vi "运维调试_古田户外.vi"() -> ()   [LabVIEW 2016]
uses:
  <vilib>/Utility/miscctls.llb/LVPointTypeDef.ctl
  PLC/PLC.lvlib
panel:
  in  "运维调试单选按钮":T1(xcontrol)
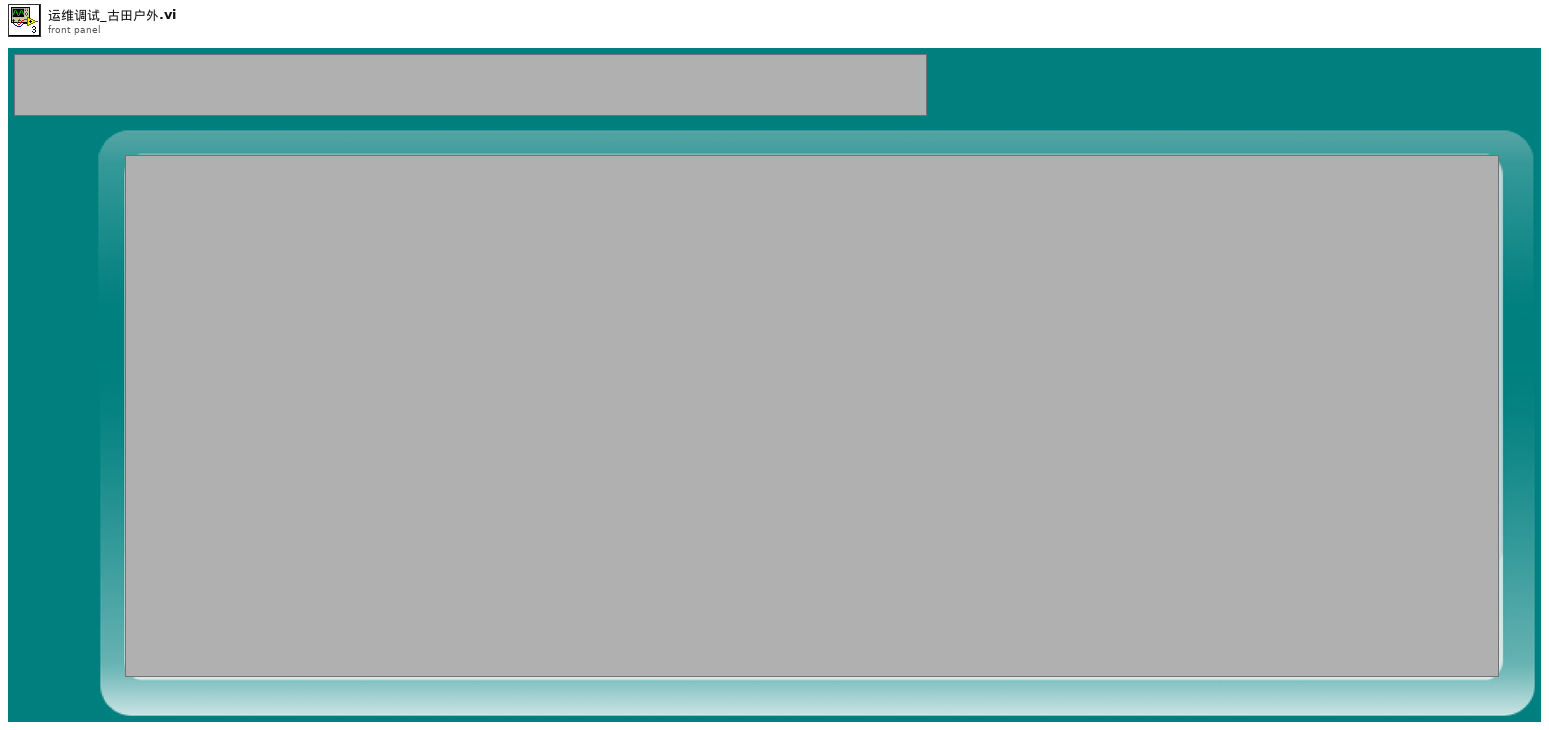
[diagram p1: front panel]
types:
  T1 = enum16{"采配水", "CODmn", "总磷氨氮", "多参数", "质控单元", "其他"}
  T2 = typedef "LVPointTypeDef.ctl" = cluster{"Horizontal":i16, "Vertical":i16}
  T3 = enum32{"Bad", "Idle", "Run top level", "Running"}
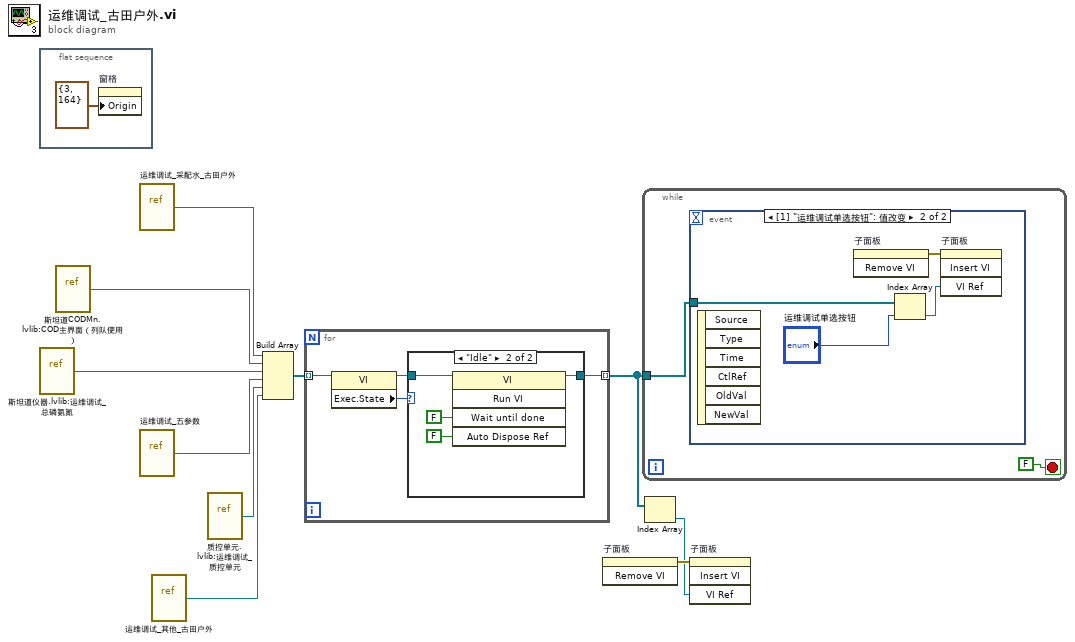
[diagram p0: block diagram]
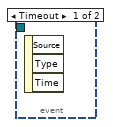
[diagram p3: hidden frame]
diagram:
  n1 = flat-sequence {
    frame #0 {
      n2 = property on="窗格" class="Pane"("Origin"=T2 {"Horizontal"=3, "Vertical"=164} ("原点")) -> ()  [unwired: 2 in, 2 out]
    }
  }
  n3 = vi-ref "斯坦道仪器.lvlib:运维调试_总磷氨氮.vi"() -> (w3:refnum<vi>)
  n4 = vi-ref "斯坦道CODMn.lvlib:COD主界面（列队使用）.vi"() -> (w4:refnum<vi>)
  n5 = vi-ref "运维调试_采配水_古田户外.vi"() -> (w7:refnum<vi>)
  n6 = vi-ref "运维调试_五参数.vi"() -> (w6:refnum<vi>)
  n7 = vi-ref "运维调试_其他_古田户外.vi"() -> (w2:refnum<vi>)
  n8 = vi-ref "质控单元.lvlib:运维调试_质控单元.vi"() -> (w1:refnum<vi>)
  n9 = Build Array(w7, w4, w3, w6, w1, w2) -> (w5:refnum<vi>[])
  n10 = for {
    tunnel: w5 -> [w15] mode=indexing
    tunnel: [w12] -> w9 mode=indexing
    n11 = property class="VI"(reference=w15) -> (reference out=w13:refnum<vi>, "Exec.State"=w14:T3)  [unwired: 1 in, 1 out]
    n12 = case shown="\"Idle\"" w14 {
      tunnel: w13 -> [w16 w18]
      tunnel: [w16 w17] -> w12
      frame "Bad", Default {
      }
      frame "Idle" {
        n13 = invoke class="VI" method="Run VI"(reference=w18, "Wait until done"=FALSE ("结束前等待"), "Auto Dispose Ref"=FALSE ("自动销毁引用")) -> (reference out=w17:refnum<vi>)  [unwired: 2 in, 4 out]
      }
    }
  }
  n14 = invoke on="子面板" class="SubPnl" method="Remove VI"() -> (error out=w10:errorcluster)  [unwired: 3 in, 2 out]
  n15 = while {
    tunnel: w9 -> [w21]
    stop <- FALSE stop-if-true
    n16 = event shown="[1] \"运维调试单选按钮\": 值改变" {
      selector: _ -> [_ _]
      dyn-events: _ -> [_ _]
      timeout: _ -> [_ _]
      tunnel: w21 -> [_ w24]
      event Timeout {
        n17 = event-data() -> ()  [unwired: 1 in, 3 out]
      }
      event "运维调试单选按钮": Value Change {
        n18 = event-data() -> ()  [unwired: 1 in, 6 out]
        n19 = invoke on="子面板" class="SubPnl" method="Remove VI"() -> (error out=w26:errorcluster)  [unwired: 3 in, 2 out]
        n20 = Index Array(array=w24, index="运维调试单选按钮") -> (element=w23:refnum<vi>)
        n21 = invoke on="子面板" class="SubPnl" method="Insert VI"(error in=w26, "VI Ref"=w23) -> ()  [unwired: 2 in, 4 out]
      }
    }
  }
  n22 = Index Array(array=w9) -> (element=w8:refnum<vi>)  [unwired: 1 in]
  n23 = invoke on="子面板" class="SubPnl" method="Insert VI"(error in=w10, "VI Ref"=w8) -> ()  [unwired: 2 in, 4 out]
